vi "Timer2.vi"(8 "error in (no error)":errorcluster, 9 "Time Target (s)":dbl=1.0, 10 "Reset":bool, 11 "Pause":bool) -> (0 "error out":errorcluster, 1 "Elapsed Time (s)":dbl, 2 "Time has Elapsed":bool)   [LabVIEW 2014]
doc: "Timer Module.\nDetermines the elapsed time using a functional global variable. The Timer has the option to restart the time and pause the count time."
panel:
  # "CONTROLS"
  # "INDICATORS"
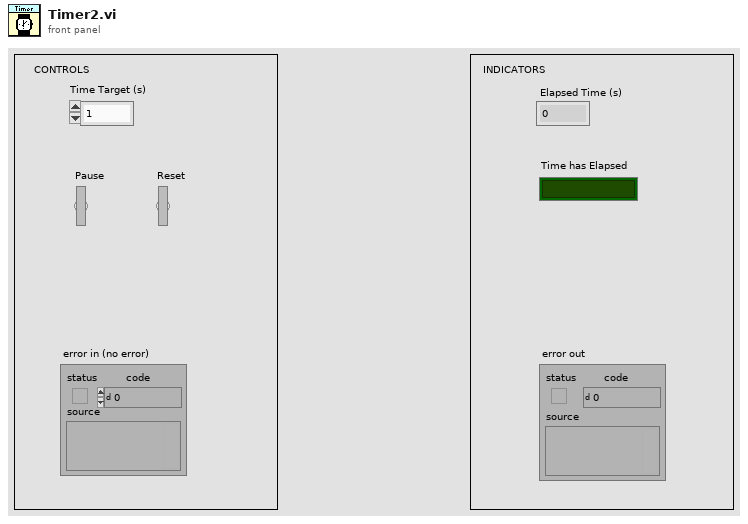
[diagram p1: front panel]
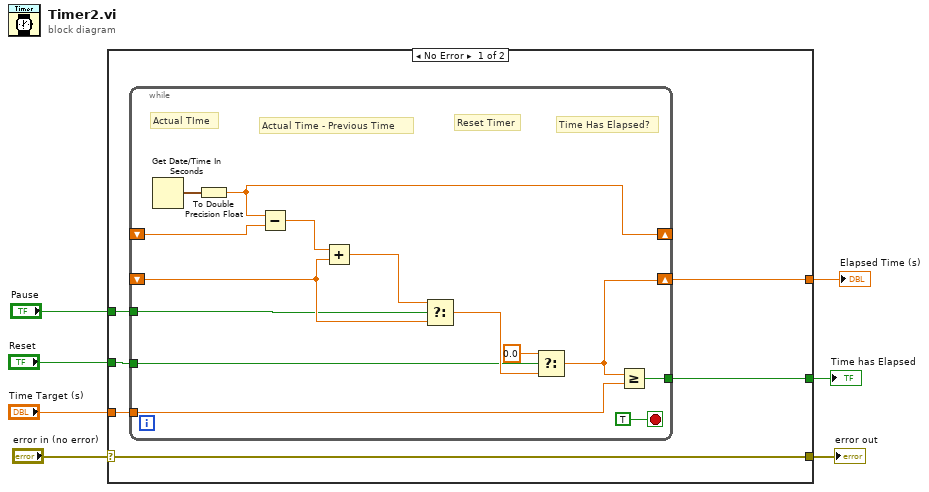
[diagram p0: block diagram]
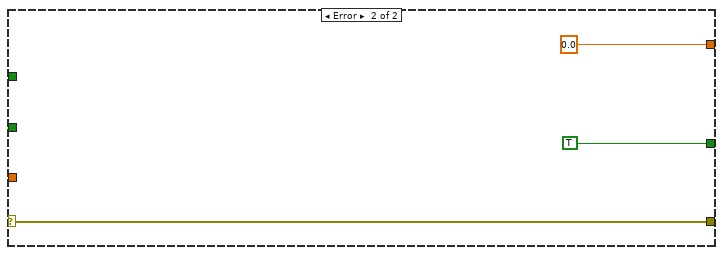
[diagram p2: hidden frame]
diagram:
  n1 = case shown="No Error" "error in (no error)" {
    selector: "error in (no error)" -> [w8 w30]
    tunnel: [w8 w30] -> w6
    tunnel: "Pause" -> [w13 _]
    tunnel: "Reset" -> [w12 _]
    tunnel: "Time Target (s)" -> [w11 _]
    tunnel: [w10 TRUE] -> w2
    tunnel: [w9 0.0 ("t")] -> w1
    frame No Error {
      n2 = while {
        shift-right: [w24] -> _
        shift-left: _ -> [w22]
        shift-right: [w14] -> w9
        shift-left: _ -> [w21]
        tunnel: w13 -> [w20]
        tunnel: w12 -> [w18]
        tunnel: w11 -> [w16]
        tunnel: [w15] -> w10
        stop <- TRUE stop-if-true
        # "Time Has Elapsed?"
        # "Reset Timer"
        # "Actual Time - Previous Time"
        # "Actual TIme"
        n3 = Get Date/Time In Seconds() -> (seconds since 1Jan1904=w26:timestamp)
        n4 = To Double Precision Float(number=w26) -> (double precision float=w24:dbl)
        n5 = Subtract(x=w24, y=w22) -> (x-y=w25:dbl)
        n6 = Add(x=w25, y=w21) -> (x+y=w23:dbl)
        n7 = Select(t=w23, s=w20, f=w21) -> (s? t:f=w19:dbl)
        n8 = Select(t=0.0, s=w18, f=w19) -> (s? t:f=w14:dbl)
        n9 = Greater Or Equal?(x=w14, y=w16) -> (x >= y?=w15:bool)
      }
    }
    frame Error {
    }
  }
  "error out" <- w6
  "Time has Elapsed" <- w2
  "Elapsed Time (s)" <- w1
